vi "LVAPT-GIT-Commit.vi"(11 "path":path) -> ()   [LabVIEW 2019]
uses:
  <vilib>/Hampel Software Engineering/Git API/Git API/GIT-api.lvclass/GIT-api.ctl
  <vilib>/Hampel Software Engineering/Git API/Git API/Accessors/GIT-Set Working Dir.vi
  <vilib>/Hampel Software Engineering/Git API/Git API/GIT-api.lvclass
panel:
  out "Staged Files":string[](array[string])
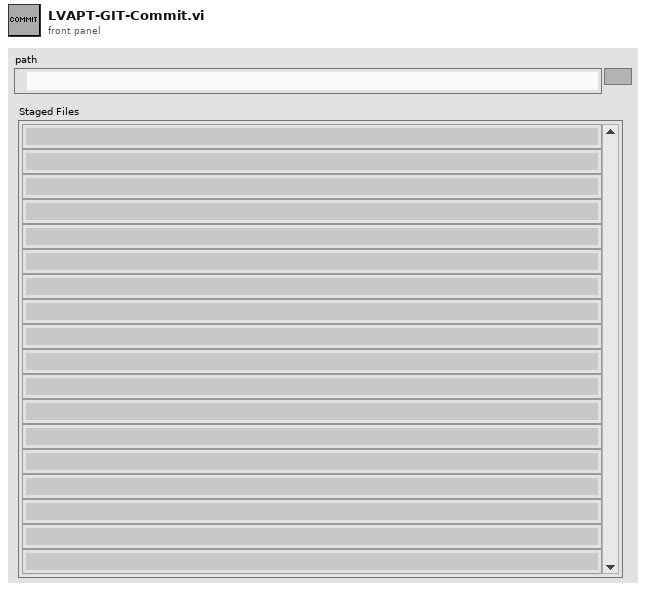
[diagram p1: front panel]
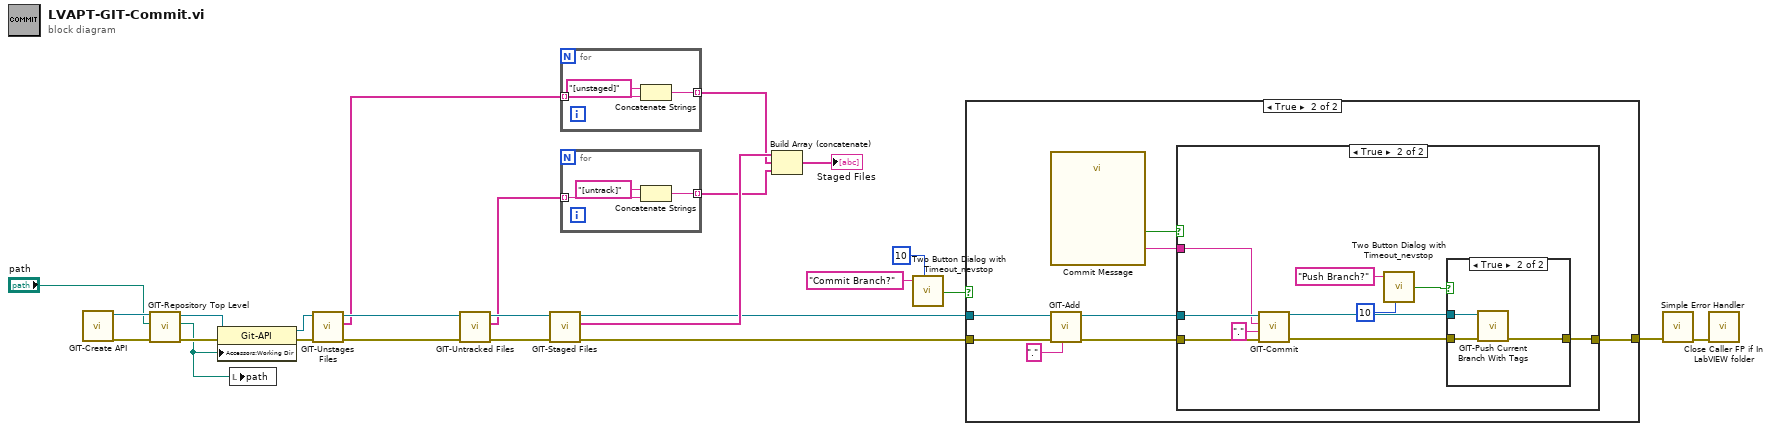
[diagram p0: block diagram]
diagram:
  n1 = call <vilib>:"GIT-Create API.vi"() -> ("error out"=w22:errorcluster, "git-api out"=w23:refnum<class "GIT-api.lvclass">)  [unwired: 10 in]
  n2 = call <vilib>:"GIT-Repository Top Level.vi"("error in"=w22, "Current Path"="path", "git-api in"=w23) -> ("error out"=w25:errorcluster, "Repo Top Level Path"=w18:path, "git-api out"=w24:refnum<class "GIT-api.lvclass">)  [unwired: 6 in]
  n3 = property class="Git-API"(reference=w24, error in=w25, "Accessors:Working Dir"=w18) -> (reference out=w6:refnum<class "GIT-api.lvclass">, error out=w7:errorcluster)
  n4 = local write "path"(w18) -> ()
  n5 = call <vilib>:"GIT-Unstages Files.vi"("error in"=w7, "Git-API in"=w6) -> ("error out"=w15:errorcluster, "Unstaged Files"=w12:string[], "Git-API out"=w16:refnum<class "GIT-api.lvclass">)  [unwired: 7 in]
  n6 = call <vilib>:"GIT-Untracked Files.vi"("error in"=w15, "Git-API in"=w16) -> ("error out"=w14:errorcluster, "Untracked Files"=w11:string[], "Git-API out"=w13:refnum<class "GIT-api.lvclass">)  [unwired: 7 in]
  n7 = call <vilib>:"GIT-Staged Files.vi"("error in"=w14, "Git-API in"=w13) -> ("error out"=w5:errorcluster, "Staged Files"=w17:string[], "Git-API out"=w4:refnum<class "GIT-api.lvclass">)  [unwired: 7 in]
  n8 = for {
    tunnel: w12 -> [w28] mode=indexing
    tunnel: [w26] -> w9 mode=indexing
    n9 = Concatenate Strings("[unstaged]" ("string"), w28) -> (w26:string)
  }
  n10 = for {
    tunnel: w11 -> [w31] mode=indexing
    tunnel: [w29] -> w8 mode=indexing
    n11 = Concatenate Strings("[untrack]" ("string"), w31) -> (w29:string)
  }
  n12 = Build Array (concatenate)(w17, w9, w8) -> (→"Staged Files":string[])
  n13 = call <userlib>:"Two Button Dialog with Timeout_nevstop.vi"("message"="Commit Branch?", "T Timeout(-1 s)"=10 ("F Timeout(-1 s)")) -> ("T button?"=w2:bool)  [unwired: 3 in]
  n14 = case shown="True" w2 {
    tunnel: [w32 w38] -> w20
    tunnel: w4 -> [_ w36]
    tunnel: w5 -> [w32 w35]
    frame False {
    }
    frame True {
      n15 = call "Commit Message"() -> ("Message"=w40:string, "OK"=w39:bool)  [unwired: 17 in, 1 out]
      n16 = call <vilib>:"GIT-Add.vi"("param"=".", "error in"=w35, "git-api in"=w36) -> ("error out"=w34:errorcluster, "git-api out"=w33:refnum<class "GIT-api.lvclass">)  [unwired: 6 in, 1 out]
      n17 = case shown="True" w39 {
        tunnel: [w41 w46] -> w38
        tunnel: w33 -> [_ w51]
        tunnel: w34 -> [w41 w50]
        tunnel: w40 -> [_ w48]
        frame False {
        }
        frame True {
          n18 = call <vilib>:"GIT-Commit.vi"("error in"=w50, "params"=".", "msg"=w48, "Git-API in"=w51) -> ("error out"=w47:errorcluster, "Git-API out"=w45:refnum<class "GIT-api.lvclass">)  [unwired: 6 in]
          n19 = call <userlib>:"Two Button Dialog with Timeout_nevstop.vi"("message"="Push Branch?", "F Timeout(-1 s)"=10) -> ("T button?"=w42:bool)  [unwired: 3 in]
          n20 = case shown="True" w42 {
            tunnel: w47 -> [w52 w55]
            tunnel: [w52 w54] -> w46
            tunnel: w45 -> [_ w53]
            frame False {
            }
            frame True {
              n21 = call <vilib>:"GIT-Push Current Branch With Tags.vi"("error in"=w55, "Git-API in"=w53) -> ("error out"=w54:errorcluster)  [unwired: 8 in, 1 out]
            }
          }
        }
      }
    }
  }
  n22 = call <vilib>:"Simple Error Handler.vi"("error in (no error)"=w20) -> ("error out"=w19:errorcluster)  [unwired: 4 in, 4 out]
  n23 = call "Close Caller FP if In LabVIEW folder.vi"("error in (no error)"=w19) -> ()  [unwired: 10 in, 1 out]
